vi "Test_SI656.vi"() -> ()   [LabVIEW 2022 SP3]
uses:
  SI_modules/SI656/SI656.lvclass
panel:
  out "% PG":cluster{"Time":timestamp[], dbl[]}(graph)
  out "Inputs":cluster{"Time":timestamp[], dbl[]}[](graph)
  out "Outputs":cluster{"Time":timestamp[], dbl[]}[](graph)
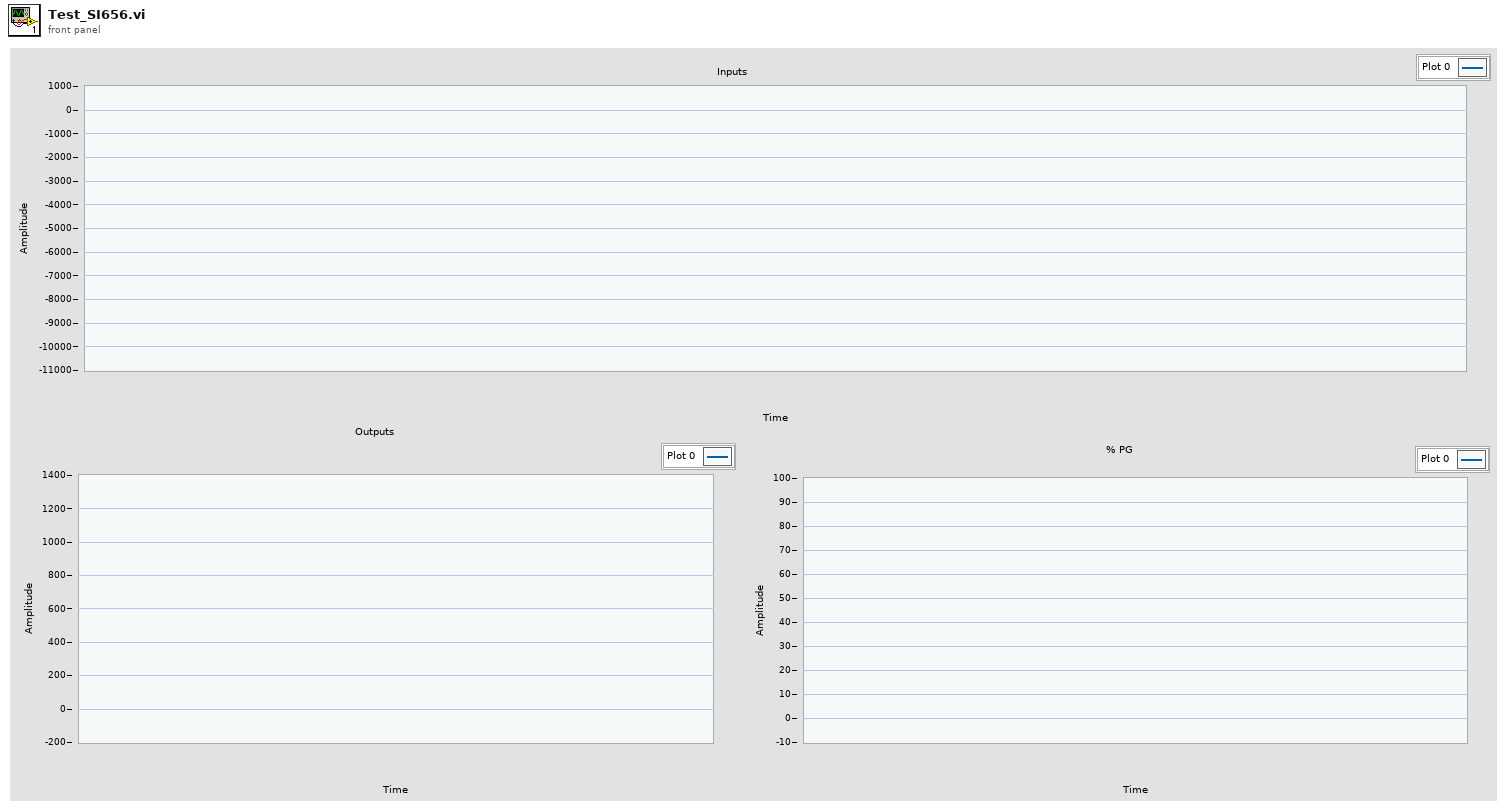
[diagram p1: front panel]
types:
  T1 = cluster{"[0]":cluster{"Time":timestamp[], "KKS":string, "Meas":dbl[]}, "[1]":cluster{"Time":timestamp[], "KKS":string, "Meas":dbl[]}, "[2]":cluster{"Time":timestamp[], "KKS":string, "Meas":dbl[]}, "[3]":cluster{"Time":timestamp[], "KKS":string, "Meas":dbl[]}, "[4]":cluster{"Time":timestamp[], "KKS":string, "Meas":dbl[]}, "[5]":cluster{"Time":timestamp[], "KKS":string, "Meas":dbl[]}, "[6]":cluster{"Time":timestamp[], "KKS":string, "Meas":dbl[]}, "[7]":cluster{"Time":timestamp[], "KKS":string, "Meas":dbl[]}, "[8]":cluster{"Time":timestamp[], "KKS":string, "Meas":dbl[]}}
  T2 = cluster{"AO1":dbl, "AO1":dbl, "AO1":dbl, "AO1":dbl}
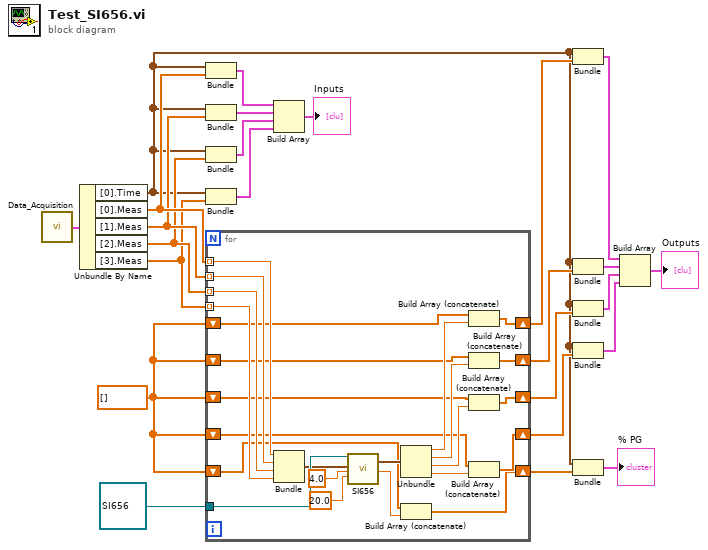
[diagram p0: block diagram]
diagram:
  w4 = dbl[] []
  n1 = call "Data_Acquisition.vi"() -> ("Meas"=w23:T1)  [unwired: 15 in]
  n2 = Unbundle By Name(w23) -> ("[0].Time"=w2:timestamp[], "[0].Meas"=w13:dbl[], "[1].Meas"=w12:dbl[], "[2].Meas"=w11:dbl[], "[3].Meas"=w10:dbl[])
  n3 = Bundle("Time"=w2, "Meas"=w13) -> (w9:cluster{"Time":timestamp[], "Meas":dbl[]})  [unwired: 1 in]
  n4 = Bundle("Time"=w2, "Meas"=w12) -> (w8:cluster{"Time":timestamp[], "Meas":dbl[]})  [unwired: 1 in]
  n5 = Bundle("Time"=w2, "Meas"=w11) -> (w7:cluster{"Time":timestamp[], "Meas":dbl[]})  [unwired: 1 in]
  n6 = Bundle("Time"=w2, "Meas"=w10) -> (w6:cluster{"Time":timestamp[], "Meas":dbl[]})  [unwired: 1 in]
  n7 = for {
    tunnel: refnum<class "SI656.lvclass"> refnum ("SI656 in") -> [w48]
    tunnel: w13 -> [w45] mode=indexing
    tunnel: w12 -> [w44] mode=indexing
    tunnel: w11 -> [w43] mode=indexing
    tunnel: w10 -> [w42] mode=indexing
    shift-right: [w39] -> w22
    shift-left: w4 -> [w35]
    shift-right: [w38] -> w21
    shift-left: w4 -> [w32]
    shift-right: [w37] -> w20
    shift-left: w4 -> [w31]
    shift-right: [w36] -> w19
    shift-left: w4 -> [w29]
    shift-right: [w26] -> w3
    shift-left: w4 -> [w25]
    n8 = Bundle(w45, w44, w43, w42) -> (w41:cluster{dbl, dbl, dbl, dbl})  [unwired: 1 in]
    n9 = call "SI656.vi"("SI656 in"=w48, "From Turbine"=w41, "In1"=4.0, "In2"=20.0) -> ("output for testing"=w40:T2, "PG 2nd Min in %"=w27:dbl)  [unwired: 11 in, 3 out]
    n10 = Unbundle(w40) -> ("AO1"=w34:dbl, "AO1"=w33:dbl, "AO1"=w30:dbl, "AO1"=w28:dbl)
    n11 = Build Array (concatenate)(w25, w27) -> (w26:dbl[])
    n12 = Build Array (concatenate)(w35, w34) -> (w39:dbl[])
    n13 = Build Array (concatenate)(w32, w33) -> (w38:dbl[])
    n14 = Build Array (concatenate)(w31, w30) -> (w37:dbl[])
    n15 = Build Array (concatenate)(w29, w28) -> (w36:dbl[])
  }
  n16 = Build Array(w9, w8, w7, w6) -> (→"Inputs":cluster{"Time":timestamp[], "Meas":dbl[]}[])
  n17 = Bundle("Time"=w2, w22) -> (w18:cluster{"Time":timestamp[], dbl[]})  [unwired: 1 in]
  n18 = Bundle("Time"=w2, w21) -> (w17:cluster{"Time":timestamp[], dbl[]})  [unwired: 1 in]
  n19 = Bundle("Time"=w2, w20) -> (w16:cluster{"Time":timestamp[], dbl[]})  [unwired: 1 in]
  n20 = Bundle("Time"=w2, w19) -> (w15:cluster{"Time":timestamp[], dbl[]})  [unwired: 1 in]
  n21 = Bundle("Time"=w2, w3) -> (→"% PG":cluster{"Time":timestamp[], dbl[]})  [unwired: 1 in]
  n22 = Build Array(w18, w17, w16, w15) -> (→"Outputs":cluster{"Time":timestamp[], dbl[]}[])
